vi "动态时间的规整.vi"(1 "参考模板特征":dbl[][](array[numeric]) format="%.2f", 2 "测试模板特征":dbl[][](array[numeric]) format="%.2f") -> ()   [LabVIEW 2018]
panel:
  out "错误输出 3":errorcluster caption="错误输出"
  out "说话人序号 2":dbl
  out "似然距离 2":dbl
  out "似然估计":dbl[](array[numeric])
  out "sigma大小":i32[](array[numeric])
  out "sigma行数":dbl
  out "输入sigma大小":dbl[](array[numeric])
  out "输入sigma":dbl[][](array[numeric]) format="%#_13g"
  out "错误输出":errorcluster
  in  "sigma":dbl[][](array[numeric]) format="%#_13g"
  in  "pai":dbl[](array[numeric]) format="%#_13g"
  in  "mu":dbl[][](array[numeric]) format="%#_13g"
  out "k":i32
  out "sigma大小":i32[](array[numeric])
  in  "cof":dbl[][](array[numeric])
  out "MU":i32[](array[numeric])
  out "X COF":i32[](array[numeric])
  out "滤波后":dbl[][](graph)
  out "待识别语音":dbl[][](graph)
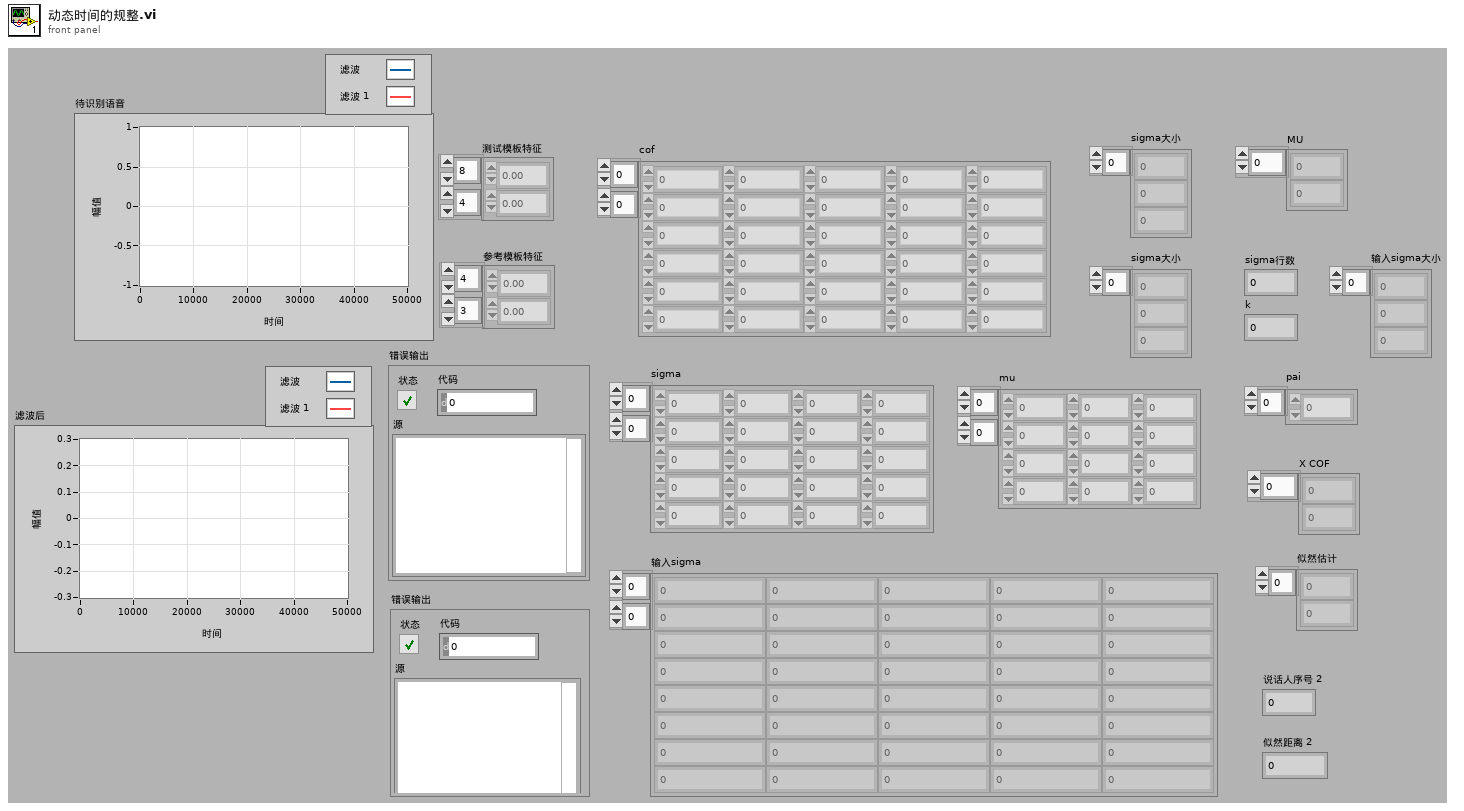
[diagram p1: front panel]
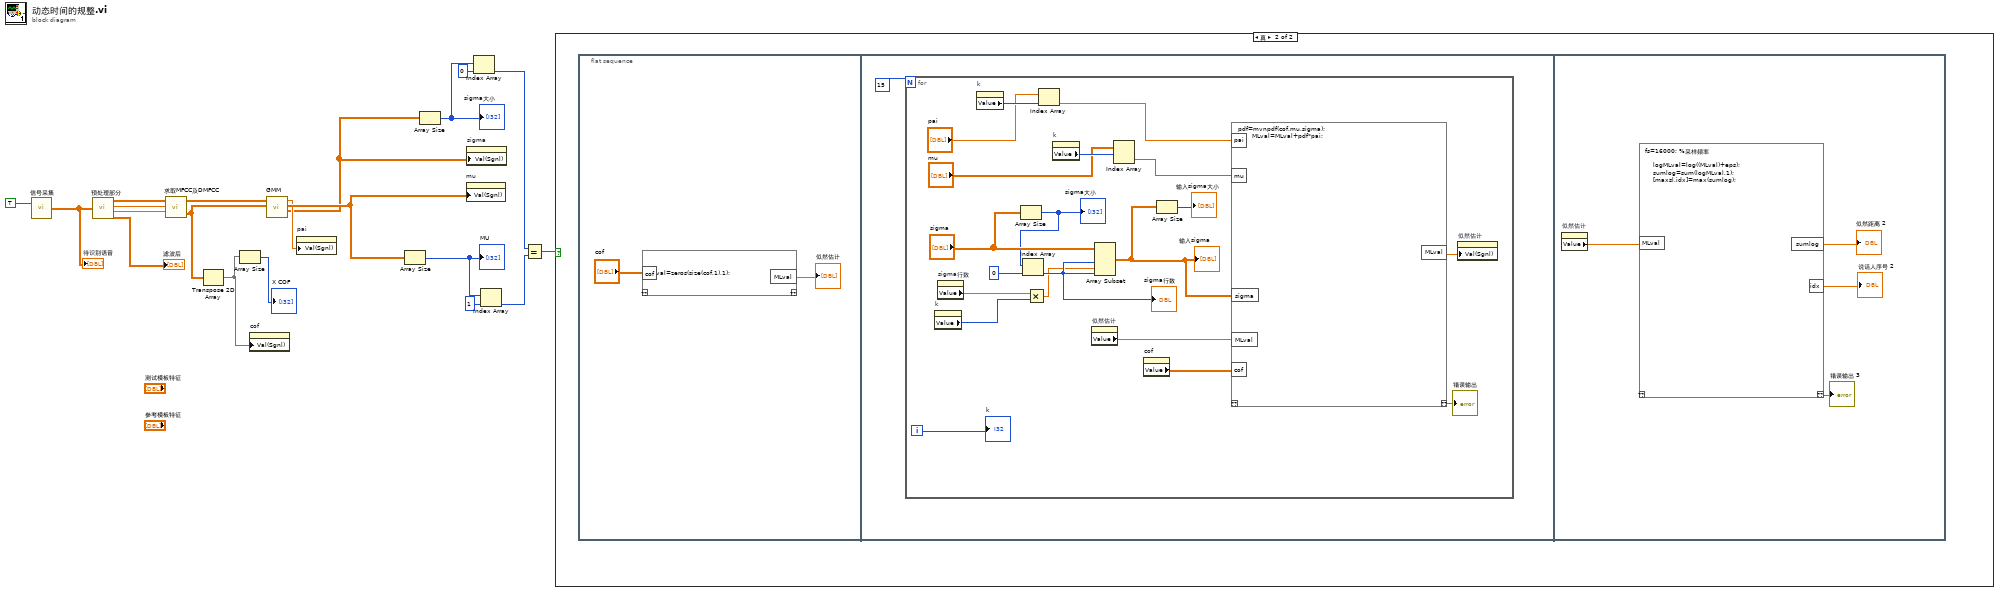
[diagram p0: block diagram]
diagram:
  n1 = call "信号采集.vi"("Boolean"=TRUE) -> ("mono 16-bit"=w16:dbl[][])  [unwired: 1 in]
  "待识别语音" <- w16
  n2 = call "预处理部分.vi"("mono 16-bit"=w16) -> ("y"=w20:dbl[][], "s1"=w19:dbl, "s2"=w18:dbl, "波形图 2"=→"滤波后":dbl[][])
  n3 = call "求取MFCC及DMFCC.vi"("s2"=w18, "s1"=w19, "xx"=w20) -> ("cof"=w10:dbl[][], "ccc"=w14:dbl[][])
  n4 = Transpose 2D Array(2D array=w10) -> (transposed array=w2:dbl[][])
  n5 = Array Size(array=w2) -> (size(s)=→"X COF":i32[])
  n6 = property on="cof" class="Arr (严格)"("Val(Sgnl)"=w2) -> ()  [unwired: 2 in, 2 out]
  n7 = call "GMM.vi"("cof"=w10, "cc"=w14) -> ("sigema"=w1:dbl[][], "mu"=w12:dbl[][], "pai"=w11:dbl[])  [unwired: 6 in]
  n8 = property on="pai" class="Arr (严格)"("Val(Sgnl)"=w11) -> ()  [unwired: 2 in, 2 out]
  n9 = Array Size(array=w12) -> (size(s)=w5:i32[])
  "MU" <- w5
  n10 = Array Size(array=w1) -> (size(s)=w9:i32[])
  "sigma大小" <- w9
  n11 = property on="mu" class="Arr (严格)"("Val(Sgnl)"=w12) -> ()  [unwired: 2 in, 2 out]
  n12 = property on="sigma" class="Arr (严格)"("Val(Sgnl)"=w1) -> ()  [unwired: 2 in, 2 out]
  n13 = Index Array(array=w9, index=0 ("索引")) -> (element=w6:i32)
  n14 = Index Array(array=w5, index=1 ("索引")) -> (element=w3:i32)
  n15 = Equal?(x=w6, y=w3) -> (x = y?=w7:bool)
  n16 = case shown="真" w7 {
    frame False {
    }
    frame True {
      n17 = flat-sequence {
        frame #0 {
          n18 = script code="MLval=zeros(size(cof,1),1);"("cof"="cof") -> ("MLval"=→"似然估计":dbl[])  [unwired: 1 in, 1 out]
        }
        frame #1 {
          n19 = for {
            N: 15 -> [_]
            i -> [w33]
            n20 = property on="k" class="DigNum (严格)"() -> ("Value"=w35:i32)  [unwired: 2 in, 2 out]
            n21 = property on="sigma行数" class="DigNum (严格)"() -> ("Value"=w41:dbl)  [unwired: 2 in, 2 out]
            n22 = property on="k" class="DigNum (严格)"() -> ("Value"=w32:i32)  [unwired: 2 in, 2 out]
            n23 = Array Size(array="sigma") -> (size(s)=w37:i32[])
            "sigma大小" <- w37
            n24 = Index Array(array=w37, index=0 ("索引")) -> (element=w42:i32)
            "sigma行数" <- w42
            n25 = Multiply(x=w41, y=w35) -> (x*y=w36:dbl)
            n26 = Index Array(array="pai", index=w32) -> (element=w30:dbl)
            n27 = property on="k" class="DigNum (严格)"() -> ("Value"=w29:i32)  [unwired: 2 in, 2 out]
            n28 = property on="似然估计" class="Arr (严格)"() -> ("Value"=w24:dbl[])  [unwired: 2 in, 2 out]
            n29 = Array Subset(array="sigma", length (row)=w42, index (col)=w36, length (col)=w42) -> (w34:dbl[][])  [unwired: 1 in]
            "输入sigma" <- w34
            n30 = Index Array(array="mu", index (row)=w29) -> (element=w27:dbl[])  [unwired: 1 in]
            n31 = property on="cof" class="Arr (严格)"() -> ("Value"=w26:dbl[][])  [unwired: 2 in, 2 out]
            n32 = Array Size(array=w34) -> (size(s)=→"输入sigma大小":i32[])
            n33 = script code="pdf=mvnpdf(cof,mu,sigma);\n       MLval=MLval+pdf*pai;"("pai"=w30, "mu"=w27, "sigma"=w34, "cof"=w26, "MLval"=w24) -> ("??"=→"错误输出":errorcluster, "MLval"=w25:dbl[])  [unwired: 1 in]
            n34 = property on="似然估计" class="Arr (严格)"("Val(Sgnl)"=w25) -> ()  [unwired: 2 in, 2 out]
            "k" <- w33
          }
        }
        frame #2 {
          n35 = property on="似然估计" class="Arr (严格)"() -> ("Value"=w44:dbl[])  [unwired: 2 in, 2 out]
          n36 = script code="fs=16000; %采样频率\n\n    logMLval=log((MLval)+eps);\n    sumlog=sum(logMLval,1);\n    [maxsl,idx]=max(sumlog);"("MLval"=w44) -> ("??"=→"错误输出 3":errorcluster, "sumlog"=→"似然距离 2":dbl, "idx"=→"说话人序号 2":dbl)  [unwired: 1 in]
        }
      }
    }
  }
